vi "Open Front Panel.vi"(6 "Custom Size":cluster{"Height":i16, "Width":i16}, 8 "error in (no error)":errorcluster, 9 "Custom Position":cluster{"Top":i16, "Left":i16}, 10 "Position":T1, 11 "IViewable in":refnum<class "IViewable.lvclass">) -> (0 "error out":errorcluster, 3 "IViewable out":refnum<class "IViewable.lvclass">)   [LabVIEW 2015, in "IViewable.lvlib" / "IViewable.lvclass"]
doc: "<License>\nCopyright © 2017 Composed Systems, LLC | All rights reserved\nwww.composed.io\n\nAuthor: Ethan Stern <ethan.stern@composed.io>\n\nThis software is provided \"AS IS\" WITHOUT WARRANTIES, either express or implied, AND IS FOR EDUCATIONAL PURPOSES ONLY.\n</License>"
uses:
  IViewable.lvclass
  View Position Enum.ctl
  IViewable.lvclass/IViewable.ctl
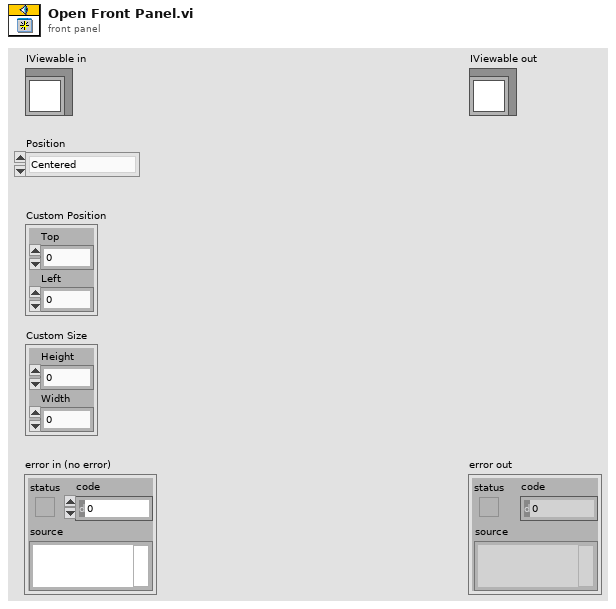
[diagram p1: front panel]
types:
  T1 = typedef "IViewable.lvlib/IViewable.lvclass/View Position Enum.ctl" = enum16{"Centered", "Maximized", "Minimized", "Custom", "Unchanged"}
  T2 = enum32{"Invalid", "Standard", "Closed", "Hidden", "Minimized", "Maximized"}
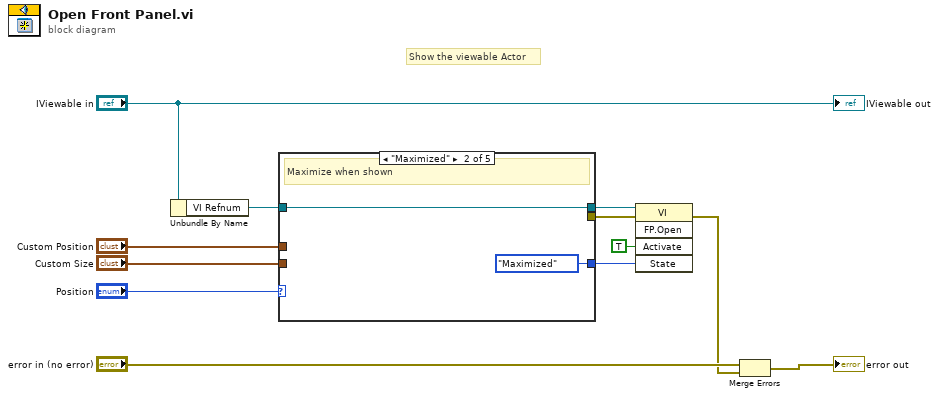
[diagram p0: block diagram]
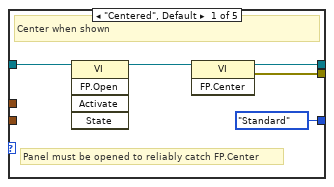
[diagram p2: hidden frame]
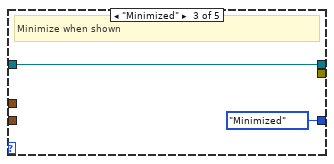
[diagram p3: hidden frame]
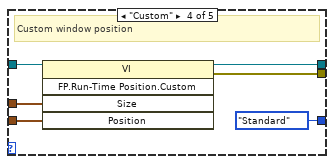
[diagram p4: hidden frame]
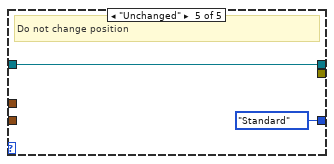
[diagram p5: hidden frame]
diagram:
  # "Show the viewable Actor"
  n1 = Unbundle By Name("IViewable in") -> ("VI Refnum"=w9:refnum<vi>)
  n2 = case shown="\"Maximized\"" "Position" {
    tunnel: w9 -> [w17 w19 w21 w27 w29]
    tunnel: [w16 w19 w21 w26 w29] -> w1
    tunnel: [w15 _ _ w25 _] -> w5
    tunnel: "Custom Position" -> [_ _ _ w24 _]
    tunnel: [T2."Standard" ("State") T2."Maximized" ("State") T2."Minimized" ("State") T2."Standard" ("State") T2."Standard" ("State")] -> w3
    tunnel: "Custom Size" -> [_ _ _ w22 _]
    frame "Centered", Default {
      # "Panel must be opened to reliably catch FP.Center"
      # "Center when shown"
      n3 = invoke class="VI" method="FP.Open"(reference=w17) -> (reference out=w13:refnum<vi>)  [unwired: 4 in, 4 out]
      n4 = invoke class="VI" method="FP.Center"(reference=w13) -> (reference out=w16:refnum<vi>, error out=w15:errorcluster)  [unwired: 2 in, 1 out]
    }
    frame "Maximized" {
      # "Maximize when shown"
    }
    frame "Minimized" {
      # "Minimize when shown"
    }
    frame "Custom" {
      # "Custom window position"
      n5 = invoke class="VI" method="FP.Run-Time Position.Custom"(reference=w27, "Size"=w24, "Position"=w22) -> (reference out=w26:refnum<vi>, error out=w25:errorcluster)  [unwired: 2 in, 3 out]
    }
    frame "Unchanged" {
      # "Do not change position"
    }
  }
  n6 = invoke class="VI" method="FP.Open"(reference=w1, error in=w5, "Activate"=TRUE ("Activate?"), "State"=w3) -> (error out=w8:errorcluster)  [unwired: 1 in, 4 out]
  n7 = Merge Errors("error in (no error)", w8) -> (→"error out":errorcluster)
  "IViewable out" <- "IViewable in"
